vi "Get DLL Path.vi"(1 "isWrapperDLL (False)":bool) -> (0 "DLL Path":path)   [LabVIEW 2020, in "KEYENCE LJ-X8000A.lvlib"]
uses:
  KEYENCE LJ-X8000A.lvlib
  Constants/Strings Definitions.ctl
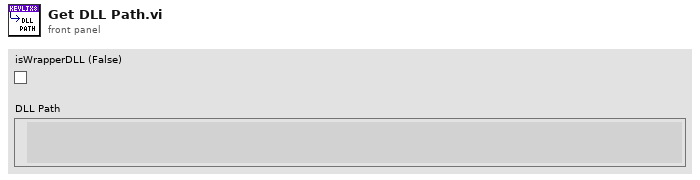
[diagram p1: front panel]
types:
  T1 = enum32{"invalid app kind", "Development System", "Run Time System", "Student Edition", "Embedded LabVIEW", "Evaluation", "Custom"}
  T2 = typedef "KEYENCE LJ-X8000A.lvlib/Strings Definitions.ctl" = string
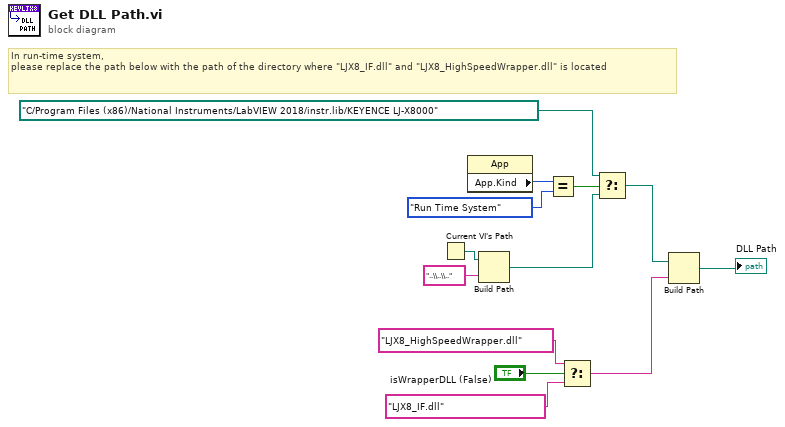
[diagram p0: block diagram]
diagram:
  # "In run-time system,\nplease replace the path below with the path of the directory where \"LJX8_IF.dll\" and \"LJX8_HighSpeedWrapper.dll\" is located"
  n1 = Current VI's Path() -> (path=w7:path)
  n2 = property class="App"() -> ("App.Kind"=w10:T1)  [unwired: 2 in, 2 out]
  n3 = Build Path(base path=w7, name or relative path="..\\..\\.." ("名前または相対パス")) -> (appended path=w4:path)
  n4 = Equal?(x=w10, y=T1."Run Time System") -> (x = y?=w8:bool)
  n5 = Select(t=T2 "LJX8_HighSpeedWrapper.dll" ("Strings Definitions"), s="isWrapperDLL (False)", f=T2 "LJX8_IF.dll" ("Strings Definitions")) -> (s? t:f=w2:T2)
  n6 = Select(t=path "C:/Program Files (x86)/National Instruments/LabVIEW 2018/instr.lib/KEYENCE LJ-X8000", s=w8, f=w4) -> (s? t:f=w3:path)
  n7 = Build Path(base path=w3, name or relative path=w2) -> (appended path=→"DLL Path":path)
